vi "GenerateAnalogWaveformPiezoTraj.vi"(8 "error in (no error)":errorcluster, 11 "SetupInfo_IN":T1={"ConfigParameters_Analog"={"JAI camera fps"=240.0, "Bi-Lateral Galvo xy scan range (V)"=0.7, "Bi-Lateral Galvo xy scan frequency (Hz)"=500, "AOM Blind percent (%)"=0.1, "AOM start blind percent (%) "=70.0, "ROI threshold"=0.5, "AO Sampling rate"=1000000.0}, "ConfigParameters_Digital"={"Steps per volume"=25.0, "Time per volume (s)"=0.4, "OG start layer"=15.0, "Objective Lin Rising Vel (micron/ms）"=1.0, "Image depth (micron)"=200.0, "OG latency (s)"=10.0, "OG repitation"=3.0, "OG end layer"=17.0, "Shock1 duration (s)"=0.001, "Shock2 duration (s)"=0.001, "Shock3 duration (s)"=0.01, "Shock4 duration (s)"=0.01, "Shock5 duration (s)"=0.1, "Shock duration_New"=[]}, "ConfigParameters_Other1"={"Frontal Galvo xy scan range (V)"=0.14, "Frontal Galvo xy scan frequency (Hz)"=500, "PFI 0 digital clock frequency"=500000.0, "Window size for layer index"=0.5, "sCMOS fps"=95.0}, "ConfigParameters_Others2"={"#Trials baseline"=6, "#Trials test"=6, "Time before acq. (s)"=360.0, "Time before test (s)"=600.0, "#Blocks acquisition"=5, "Inter-trial interval baseline (s)"=60.0, "#Trials per acquition block"=6, "Inter-block interval acquisition (s)"=360.0, "Inter-trial interval acquisition (s)"=20.0, "Flash latency (s)"=10.0, "Flash duration (s)"=3.2, "Response duration (s)"=10.0, "MaxTimeEventDetection (s)"=6, "StimType"=enum."Flash", "#MaxEvents"=6}, "ProcessParametersOut"={"stand Z vol Acquisition time (s)"=0.2631578947368421, "stand Z vol Backward time (s)"=0.13684210526315793, "Objective scan volt"=5.0, "Bi-lateral Galvo Z scan volt"=0.45, "Frontal Galvo Z scan volt"=0.37, "Objective step length (micron)"=8.0, "OG Z volet Linear Dec time (s)"=0.024, "OG Z vol Stim. steps time (s)"=0.031578947368421054, "OG Z vol Linear Acc time (s)"=0.112, "#Vol. of flash"=8, "#Vol. of shock"=1, "#Vol. bef flash"=25, "#Vol. aft flash"=17, "OG Z vol Linear Dec time (s)"=0.112, "OG Z vol time (s)"=0.39073684210526316, "Stack duration"=[0.001, 0.001, 0.01, 0.01, 0.1], "AOM stand. value size"=400000, "Plane indexing length"=0, "#Vol. blank"=0, "#Vol. blank before acq"=0, "#Vol. blank before test"=0, " #Inter-block interval acquisition (Ed-St Vol)"=0}, "WaveformParameters"={"stand Z vol Acquisition samp info"={"Fs"=1000000.0, "#s"=263158.0}, "stand Z vol Backward samp info"={"Fs"=1000000.0, "#s"=136842.0}, "OG Z vol Linear Acc samp info"={"Fs"=1000000.0, "#s"=112000.0}, "OG Z vol Stim. steps samp info"={"Fs"=1000000.0, "#s"=31579.0}, "OG Z volet Linear Dec samp info"={"Fs"=1000000.0, "#s"=24000.0}, "OG Z vol Linear Dec samp info"={"Fs"=1000000.0, "#s"=112000.0}, "OG Z vol samp info"={"Fs"=1000000.0, "#s"=390737.0}, "stand Z vol backforth samp info"={"Fs"=1000000.0, "#s"=400000.0}}, "AnalogWaveform"={"Bi-lateral Galvo Z stand waveform"={"t0"=timestamp(0 s since 1904-01-01), "dt"=1.0, "Y"=[]}, "Frontal Galvo Z stand waveform"={"t0"=timestamp(0 s since 1904-01-01), "dt"=1.0, "Y"=[]}, "Bi-lateral Galvo XY stand waveform"={"t0"=timestamp(0 s since 1904-01-01), "dt"=1.0, "Y"=[]}, "Frontal Galvo XY stand waveform"={"t0"=timestamp(0 s since 1904-01-01), "dt"=1.0, "Y"=[]}, "sCMOS stand waveform"={"t0"=timestamp(0 s since 1904-01-01), "dt"=1.0, "Y"=[]}, "Detection objective stand waveform"={"t0"=timestamp(0 s since 1904-01-01), "dt"=1.0, "Y"=[]}, "AOM stand waveform"={"t0"=timestamp(0 s since 1904-01-01), "dt"=1.0, "Y"=[]}, "PFI 0 clock stand waveform"={"t0"=timestamp(0 s since 1904-01-01), "dt"=1.0, "Y"=[]}, "Bi-lateral Galvo Z OG waveform"={"t0"=timestamp(0 s since 1904-01-01), "dt"=1.0, "Y"=[]}, "Bi-lateral Galvo XY OG waveform"={"t0"=timestamp(0 s since 1904-01-01), "dt"=1.0, "Y"=[]}, "Frontal Galvo Z OG waveform"={"t0"=timestamp(0 s since 1904-01-01), "dt"=1.0, "Y"=[]}, "Frontal Galvo XY OG waveform"={"t0"=timestamp(0 s since 1904-01-01), "dt"=1.0, "Y"=[]}, "sCMOS OG waveform"={"t0"=timestamp(0 s since 1904-01-01), "dt"=1.0, "Y"=[]}, "Detection objective OG waveform"={"t0"=timestamp(0 s since 1904-01-01), "dt"=1.0, "Y"=[]}, "AOM OG waveform"={"t0"=timestamp(0 s since 1904-01-01), "dt"=1.0, "Y"=[]}, "PFI 0 clock OG wavee"={"t0"=timestamp(0 s since 1904-01-01), "dt"=1.0, "Y"=[]}, "sCMOS blank waveform"={"t0"=timestamp(0 s since 1904-01-01), "dt"=1.0, "Y"=[]}, "All analog OG wave"=[], "All analog stand wave"=[], "All analog blank wave"=[], "BufferWaveform_Analog"=[], "Bi-lateral Galvo Z XY"={"t0"=timestamp(0 s since 1904-01-01), "dt"=1.0, "Y"=[]}, "Frontal Galvo Z XY"={"t0"=timestamp(0 s since 1904-01-01), "dt"=1.0, "Y"=[]}, "sCMOS Trigger XY"={"t0"=timestamp(0 s since 1904-01-01), "dt"=1.0, "Y"=[]}, "Detection objective XY"={"t0"=timestamp(0 s since 1904-01-01), "dt"=1.0, "Y"=[]}, "AOM XY"={"t0"=timestamp(0 s since 1904-01-01), "dt"=1.0, "Y"=[]}, "Analog_XY"=[]}, "DigitalWaveform"={"AllDigitalStandWave"=[], "AllDigialEvokedWave"=[], "AllDigialOGWave"=[], "AllDigitalPairWave_1"=[], "AllDigitalPairWave_2"=[], "AllDigitalPairWave_3"=[], "AllDigitalPairWave_4"=[], "AllDigitalPairWave_5"=[], "Plane Indexing"={"t0"=timestamp(0 s since 1904-01-01), "dt"=0.0, "Y"={"transitions"=[], "data"=[]}, "error"={"status"=FALSE, "code"=37421928, "source"=""}}, "Plane indexing P0.5 OG"={"t0"=timestamp(0 s since 1904-01-01), "dt"=0.0, "Y"={"transitions"=[], "data"=[]}, "error"={"status"=FALSE, "code"=37421928, "source"=""}}, "AllDigitalPairWaves"=[], "BufferWaveform_Digital"=[], "AllDigitalBlankWave"=[], "Digial_XY"=[], "Digital_XY_flash"=[], "Digial_XY DMD"=[]}, "PhysicalResource"={"PhysicalChannels_AI"="", "PhysicalChannels_AO"="", "PhysicalChannels_DO"="", "Task_AnalogOutput"="", "Task_DigitalOutput"="", "Task_AnalogInput"=""}, "ControlsRef"={"Mode_1"=refnum, "EventDetectionMode"=refnum, "Mode_2A"=refnum, "StimulationMode"=refnum, "Mode_2B"=refnum, "ErrorMeg"=refnum}, "test"=""} {"ConfigParameters_Other1"."Frontal Galvo xy scan frequency (Hz)" min=500 max=500; "ConfigParameters_Other1"."Frontal Galvo xy scan range (V)" min=0.0 max=1.5; "ConfigParameters_Analog"."AOM start blind percent (%)" min=10.0 max=90.0; "ConfigParameters_Analog"."AOM Blind percent (%)" min=0.1 max=100.0; "ConfigParameters_Analog"."Bi-Lateral Galvo xy scan frequency (Hz)" min=500 max=500; "ConfigParameters_Analog"."Bi-Lateral Galvo xy scan range (V)" min=0.0 max=1.5}) -> (0 "error out":errorcluster, 3 "SetupInfo_OUT":T1={"ConfigParameters_Analog"={"JAI camera fps"=240.0, "Bi-Lateral Galvo xy scan range (V)"=0.7, "Bi-Lateral Galvo xy scan frequency (Hz)"=500, "AOM Blind percent (%)"=0.1, "AOM start blind percent (%) "=70.0, "ROI threshold"=1.0, "AO Sampling rate"=1000000.0}, "ConfigParameters_Digital"={"Steps per volume"=25.0, "Time per volume (s)"=0.4, "OG start layer"=15.0, "Objective Lin Rising Vel (micron/ms）"=1.0, "Image depth (micron)"=200.0, "OG latency (s)"=10.0, "OG repitation"=3.0, "OG end layer"=17.0, "Shock1 duration (s)"=0.001, "Shock2 duration (s)"=0.001, "Shock3 duration (s)"=0.01, "Shock4 duration (s)"=0.01, "Shock5 duration (s)"=0.1, "Shock duration_New"=[]}, "ConfigParameters_Other1"={"Frontal Galvo xy scan range (V)"=0.14, "Frontal Galvo xy scan frequency (Hz)"=500, "PFI 0 digital clock frequency"=500000.0, "Window size for layer index"=0.5, "sCMOS fps"=95.0}, "ConfigParameters_Others2"={"#Trials baseline"=6, "#Trials test"=6, "Time before acq. (s)"=360.0, "Time before test (s)"=600.0, "#Blocks acquisition"=5, "Inter-trial interval baseline (s)"=60.0, "#Trials per acquition block"=6, "Inter-block interval acquisition (s)"=360.0, "Inter-trial interval acquisition (s)"=20.0, "Flash latency (s)"=10.0, "Flash duration (s)"=3.2, "Response duration (s)"=10.0, "MaxTimeEventDetection (s)"=6, "StimType"=enum."Flash", "#MaxEvents"=6}, "ProcessParametersOut"={"stand Z vol Acquisition time (s)"=0.2631578947368421, "stand Z vol Backward time (s)"=0.13684210526315793, "Objective scan volt"=5.0, "Bi-lateral Galvo Z scan volt"=0.1800000180000018, "Frontal Galvo Z scan volt"=0.14940000509752818, "Objective step length (micron)"=8.0, "OG Z volet Linear Dec time (s)"=0.024, "OG Z vol Stim. steps time (s)"=0.031578947368421054, "OG Z vol Linear Acc time (s)"=0.112, "#Vol. of flash"=8, "#Vol. of shock"=1, "#Vol. bef flash"=25, "#Vol. aft flash"=17, "OG Z vol Linear Dec time (s)"=0.112, "OG Z vol time (s)"=0.39073684210526316, "Stack duration"=[0.001, 0.001, 0.01, 0.01, 0.1], "AOM stand. value size"=400000, "Plane indexing length"=0, "#Vol. blank"=0, "#Vol. blank before acq"=0, "#Vol. blank before test"=0, " #Inter-block interval acquisition (Ed-St Vol)"=0}, "WaveformParameters"={"stand Z vol Acquisition samp info"={"Fs"=1000000.0, "#s"=263158.0}, "stand Z vol Backward samp info"={"Fs"=1000000.0, "#s"=136842.0}, "OG Z vol Linear Acc samp info"={"Fs"=1000000.0, "#s"=112000.0}, "OG Z vol Stim. steps samp info"={"Fs"=1000000.0, "#s"=31579.0}, "OG Z volet Linear Dec samp info"={"Fs"=1000000.0, "#s"=24000.0}, "OG Z vol Linear Dec samp info"={"Fs"=1000000.0, "#s"=112000.0}, "OG Z vol samp info"={"Fs"=1000000.0, "#s"=390737.0}, "stand Z vol backforth samp info"={"Fs"=1000000.0, "#s"=400000.0}}, "AnalogWaveform"={"Bi-lateral Galvo Z stand waveform"={"t0"=timestamp(0 s since 1904-01-01), "dt"=1.0, "Y"=[]}, "Frontal Galvo Z stand waveform"={"t0"=timestamp(0 s since 1904-01-01), "dt"=1.0, "Y"=[]}, "Bi-lateral Galvo XY stand waveform"={"t0"=timestamp(0 s since 1904-01-01), "dt"=1.0, "Y"=[]}, "Frontal Galvo XY stand waveform"={"t0"=timestamp(0 s since 1904-01-01), "dt"=1.0, "Y"=[]}, "sCMOS stand waveform"={"t0"=timestamp(0 s since 1904-01-01), "dt"=1.0, "Y"=[]}, "Detection objective stand waveform"={"t0"=timestamp(0 s since 1904-01-01), "dt"=1.0, "Y"=[]}, "AOM stand waveform"={"t0"=timestamp(0 s since 1904-01-01), "dt"=1.0, "Y"=[]}, "PFI 0 clock stand waveform"={"t0"=timestamp(0 s since 1904-01-01), "dt"=1.0, "Y"=[]}, "Bi-lateral Galvo Z OG waveform"={"t0"=timestamp(0 s since 1904-01-01), "dt"=1.0, "Y"=[]}, "Bi-lateral Galvo XY OG waveform"={"t0"=timestamp(0 s since 1904-01-01), "dt"=1.0, "Y"=[]}, "Frontal Galvo Z OG waveform"={"t0"=timestamp(0 s since 1904-01-01), "dt"=1.0, "Y"=[]}, "Frontal Galvo XY OG waveform"={"t0"=timestamp(0 s since 1904-01-01), "dt"=1.0, "Y"=[]}, "sCMOS OG waveform"={"t0"=timestamp(0 s since 1904-01-01), "dt"=1.0, "Y"=[]}, "Detection objective OG waveform"={"t0"=timestamp(0 s since 1904-01-01), "dt"=1.0, "Y"=[]}, "AOM OG waveform"={"t0"=timestamp(0 s since 1904-01-01), "dt"=1.0, "Y"=[]}, "PFI 0 clock OG wavee"={"t0"=timestamp(0 s since 1904-01-01), "dt"=1.0, "Y"=[]}, "sCMOS blank waveform"={"t0"=timestamp(0 s since 1904-01-01), "dt"=1.0, "Y"=[]}, "All analog OG wave"=[], "All analog stand wave"=[], "All analog blank wave"=[], "BufferWaveform_Analog"=[], "Bi-lateral Galvo Z XY"={"t0"=timestamp(0 s since 1904-01-01), "dt"=1.0, "Y"=[]}, "Frontal Galvo Z XY"={"t0"=timestamp(0 s since 1904-01-01), "dt"=1.0, "Y"=[]}, "sCMOS Trigger XY"={"t0"=timestamp(0 s since 1904-01-01), "dt"=1.0, "Y"=[]}, "Detection objective XY"={"t0"=timestamp(0 s since 1904-01-01), "dt"=1.0, "Y"=[]}, "AOM XY"={"t0"=timestamp(0 s since 1904-01-01), "dt"=1.0, "Y"=[]}, "Analog_XY"=[]}, "DigitalWaveform"={"AllDigitalStandWave"=[], "AllDigialEvokedWave"=[], "AllDigialOGWave"=[], "AllDigitalPairWave_1"=[], "AllDigitalPairWave_2"=[], "AllDigitalPairWave_3"=[], "AllDigitalPairWave_4"=[], "AllDigitalPairWave_5"=[], "Plane Indexing"={"t0"=timestamp(0 s since 1904-01-01), "dt"=0.0, "Y"={"transitions"=[], "data"=[]}, "error"={"status"=FALSE, "code"=37421928, "source"=""}}, "Plane indexing P0.5 OG"={"t0"=timestamp(0 s since 1904-01-01), "dt"=0.0, "Y"={"transitions"=[], "data"=[]}, "error"={"status"=FALSE, "code"=37421928, "source"=""}}, "AllDigitalPairWaves"=[], "BufferWaveform_Digital"=[], "AllDigitalBlankWave"=[], "Digial_XY"=[], "Digital_XY_flash"=[], "Digial_XY DMD"=[]}, "PhysicalResource"={"PhysicalChannels_AI"="", "PhysicalChannels_AO"="", "PhysicalChannels_DO"="", "Task_AnalogOutput"="", "Task_DigitalOutput"="", "Task_AnalogInput"=""}, "ControlsRef"={"Mode_1"=refnum, "EventDetectionMode"=refnum, "Mode_2A"=refnum, "StimulationMode"=refnum, "Mode_2B"=refnum, "ErrorMeg"=refnum}, "test"=""} {"ConfigParameters_Other1"."Frontal Galvo xy scan frequency (Hz)" min=500 max=500; "ConfigParameters_Other1"."Frontal Galvo xy scan range (V)" min=0.0 max=1.5; "ConfigParameters_Analog"."AOM start blind percent (%)" min=10.0 max=90.0; "ConfigParameters_Analog"."AOM Blind percent (%)" min=0.1 max=100.0; "ConfigParameters_Analog"."Bi-Lateral Galvo xy scan frequency (Hz)" min=500 max=500; "ConfigParameters_Analog"."Bi-Lateral Galvo xy scan range (V)" min=0.0 max=1.5})   [LabVIEW 2018]
uses:
  SetupInfo.ctl
  ConfigParameters_Analog.ctl
  ConfigParameters_Digital.ctl
  ConfigParameters_Others1.ctl
  ConfigParameters_Others2.ctl
  ProcessParametersOut.ctl
  WaveformParameters.ctl
  AnalogWaveform.ctl
  DigitalWaveform.ctl
  PhysicalResource.ctl
  ControlsRef.ctl
  <vilib>/Waveform/WDTOps.llb/WDT Append Waveforms DBL.vi
  <vilib>/measure/NI_MABase.lvlib
panel:
  out "piezo trajectory not in use. the trajactory version save in *copy.vi":string
  in  "FileSamplingRate":dbl=1000.0
  in  "PiezoTrajectoryPath":path=path "D:/APP/LightSheetController_Ver8 obl/VISource/Waveform/Piezo_feedback_20201106.txt"
  out "AOM stand. value size":i32=400000
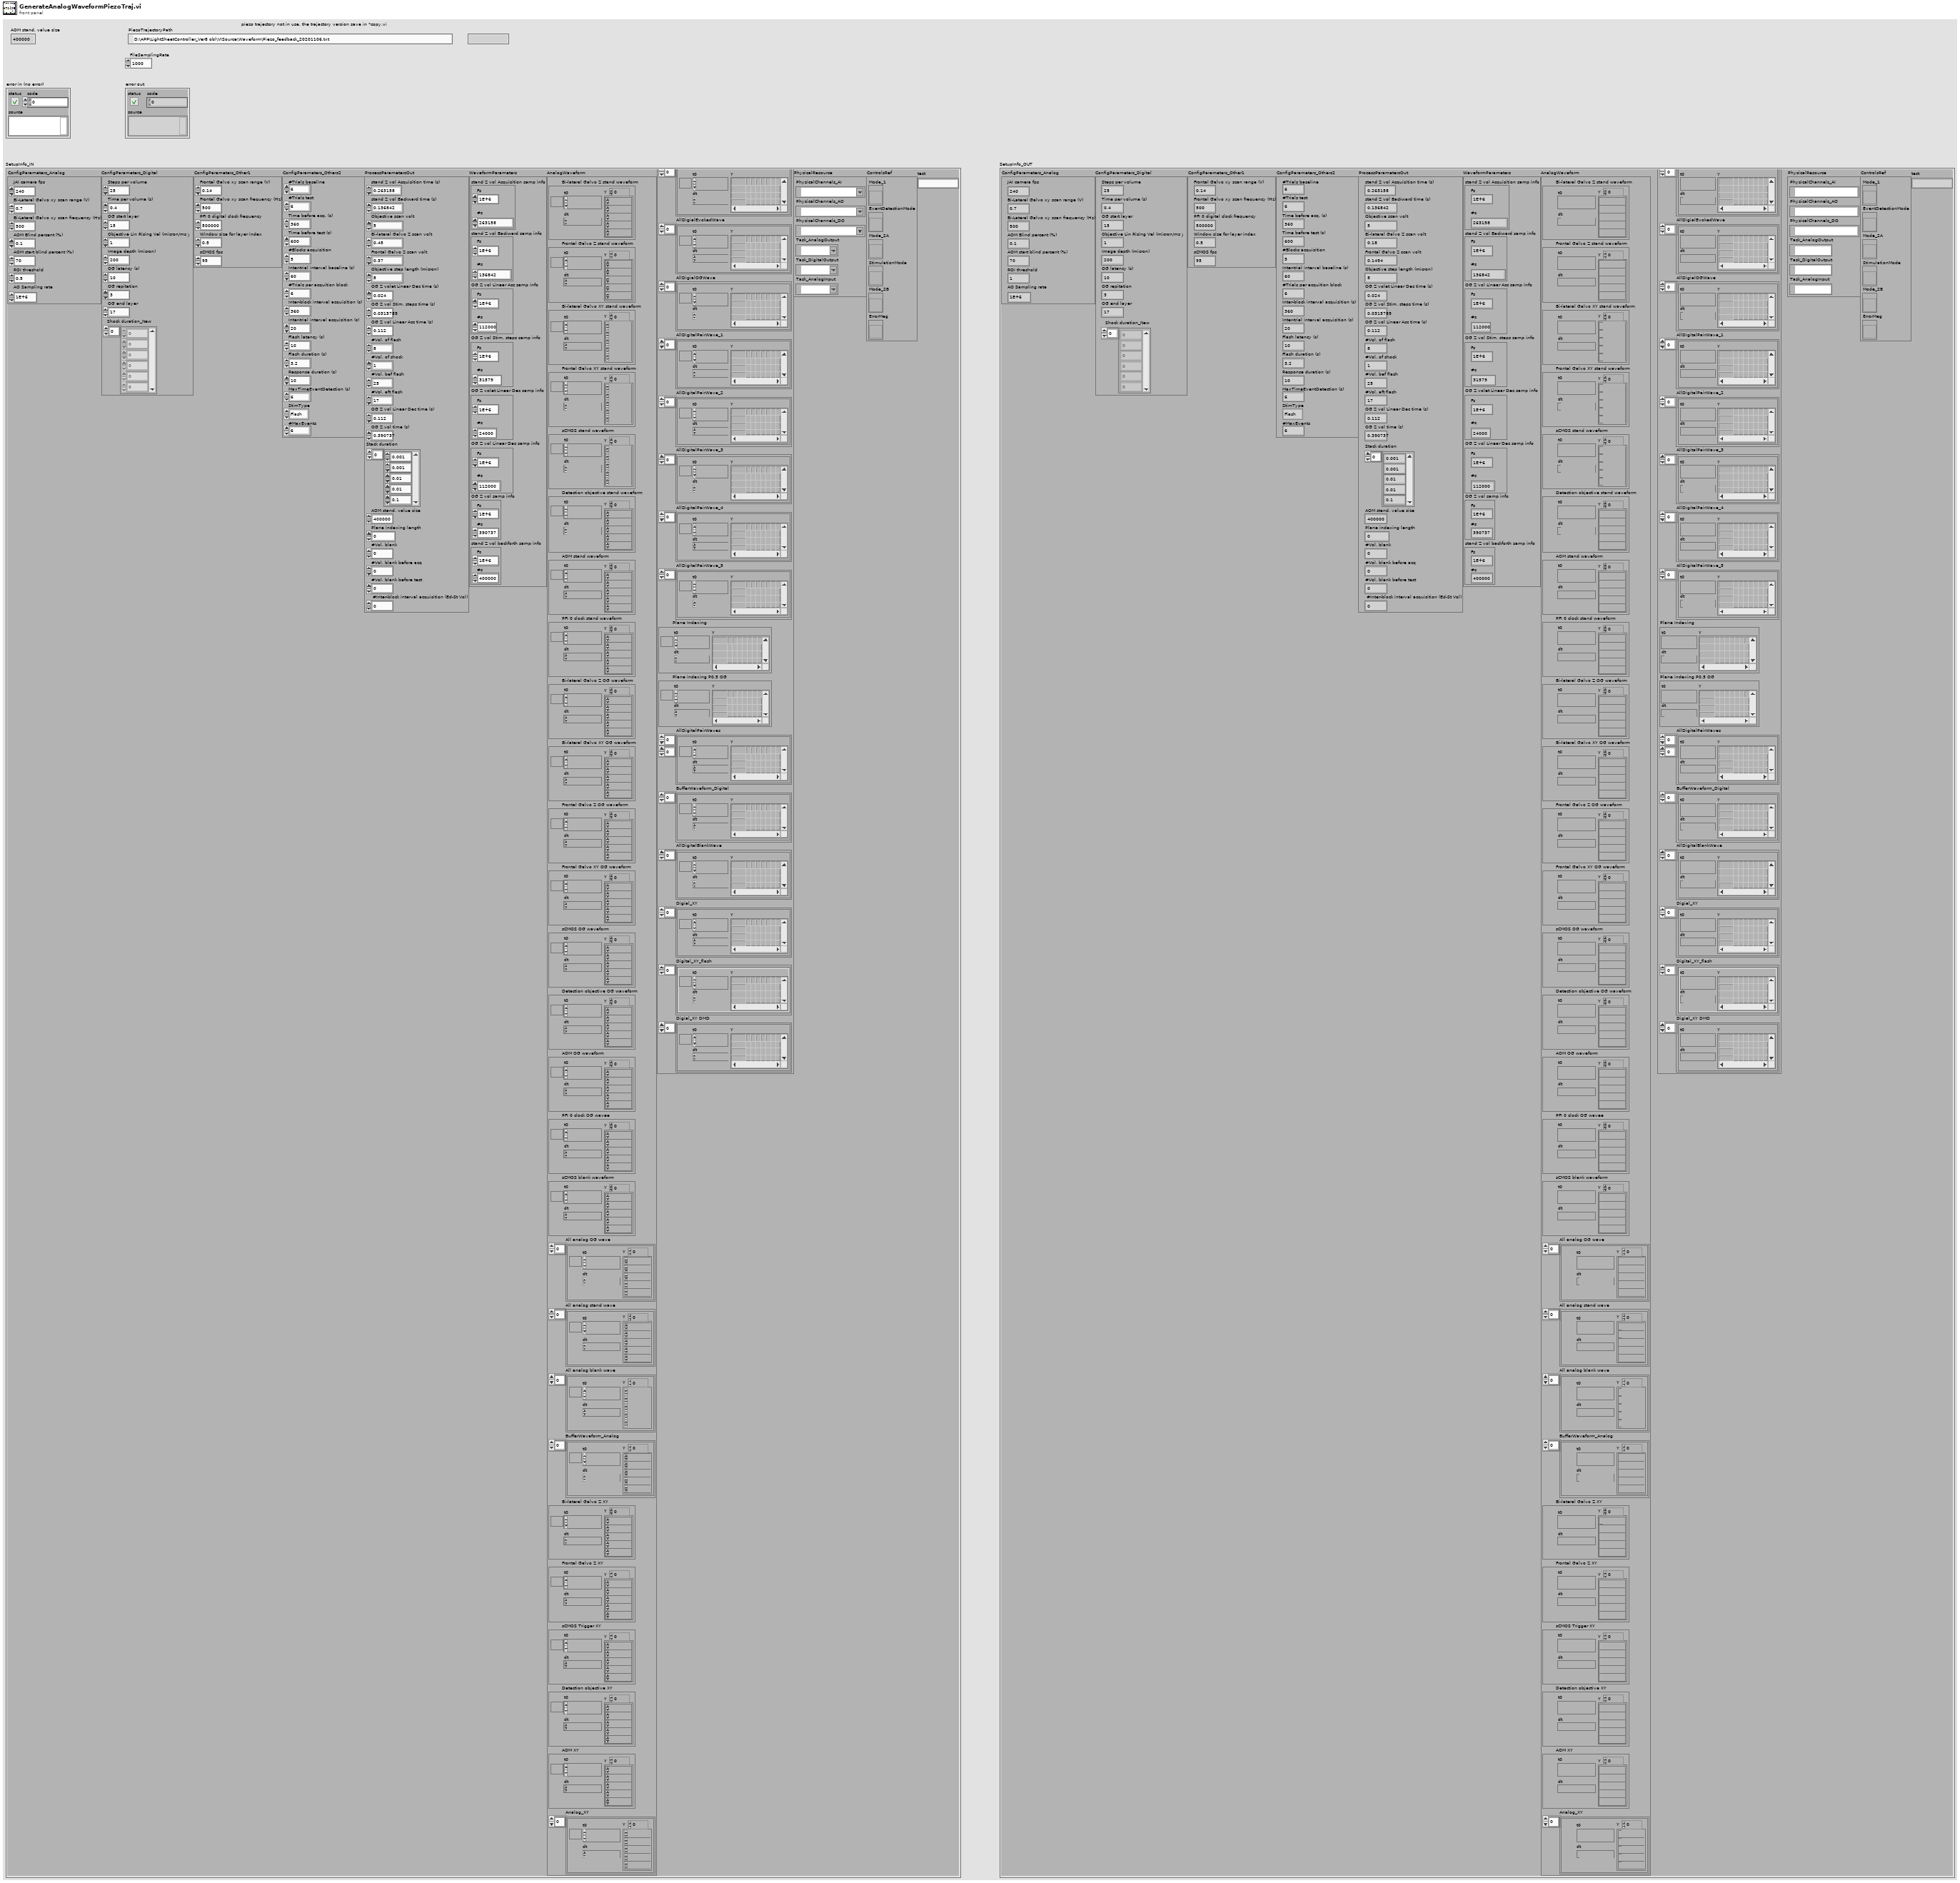
[diagram p1: front panel]
types:
  T1 = typedef "SetupInfo.ctl" = cluster{"ConfigParameters_Analog":T2, "ConfigParameters_Digital":T3, "ConfigParameters_Other1":T4, "ConfigParameters_Others2":T5, "ProcessParametersOut":T6, "WaveformParameters":T7, "AnalogWaveform":T8, "DigitalWaveform":T9, "PhysicalResource":T10, "ControlsRef":T11, "test":string}
  T2 = typedef "ConfigParameters_Analog.ctl" = cluster{"JAI camera fps":dbl, "Bi-Lateral Galvo xy scan range (V)":dbl, "Bi-Lateral Galvo xy scan frequency (Hz)":i16, "AOM Blind percent (%)":dbl, "AOM start blind percent (%) ":dbl, "ROI threshold":dbl, "AO Sampling rate":dbl}
  T3 = typedef "ConfigParameters_Digital.ctl" = cluster{"Steps per volume":dbl, "Time per volume (s)":dbl, "OG start layer":dbl, "Objective Lin Rising Vel (micron/ms）":dbl, "Image depth (micron)":dbl, "OG latency (s)":dbl, "OG repitation":dbl, "OG end layer":dbl, "Shock1 duration (s)":dbl, "Shock2 duration (s)":dbl, "Shock3 duration (s)":dbl, "Shock4 duration (s)":dbl, "Shock5 duration (s)":dbl, "Shock duration_New":dbl[]}
  T4 = typedef "ConfigParameters_Others1.ctl" = cluster{"Frontal Galvo xy scan range (V)":dbl, "Frontal Galvo xy scan frequency (Hz)":i16, "PFI 0 digital clock frequency":dbl, "Window size for layer index":dbl, "sCMOS fps":dbl}
  T5 = typedef "ConfigParameters_Others2.ctl" = cluster{"#Trials baseline":i32, "#Trials test":i32, "Time before acq. (s)":dbl, "Time before test (s)":dbl, "#Blocks acquisition":i32, "Inter-trial interval baseline (s)":dbl, "#Trials per acquition block":i32, "Inter-block interval acquisition (s)":dbl, "Inter-trial interval acquisition (s)":dbl, "Flash latency (s)":dbl, "Flash duration (s)":dbl, "Response duration (s)":dbl, "MaxTimeEventDetection (s)":i32, "StimType":enum16{"Flash", "OG"}, "#MaxEvents":i32}
  T6 = typedef "ProcessParametersOut.ctl" = cluster{"stand Z vol Acquisition time (s)":dbl, "stand Z vol Backward time (s)":dbl, "Objective scan volt":dbl, "Bi-lateral Galvo Z scan volt":dbl, "Frontal Galvo Z scan volt":dbl, "Objective step length (micron)":dbl, "OG Z volet Linear Dec time (s)":dbl, "OG Z vol Stim. steps time (s)":dbl, "OG Z vol Linear Acc time (s)":dbl, "#Vol. of flash":i32, "#Vol. of shock":i32, "#Vol. bef flash":i32, "#Vol. aft flash":i32, "OG Z vol Linear Dec time (s)":dbl, "OG Z vol time (s)":dbl, "Stack duration":dbl[], "AOM stand. value size":i32, "Plane indexing length":i32, "#Vol. blank":i32, "#Vol. blank before acq":i32, "#Vol. blank before test":i32, " #Inter-block interval acquisition (Ed-St Vol)":i32}
  T7 = typedef "WaveformParameters.ctl" = cluster{"stand Z vol Acquisition samp info":cluster{"Fs":dbl, "#s":dbl}, "stand Z vol Backward samp info":cluster{"Fs":dbl, "#s":dbl}, "OG Z vol Linear Acc samp info":cluster{"Fs":dbl, "#s":dbl}, "OG Z vol Stim. steps samp info":cluster{"Fs":dbl, "#s":dbl}, "OG Z volet Linear Dec samp info":cluster{"Fs":dbl, "#s":dbl}, "OG Z vol Linear Dec samp info":cluster{"Fs":dbl, "#s":dbl}, "OG Z vol samp info":cluster{"Fs":dbl, "#s":dbl}, "stand Z vol backforth samp info":cluster{"Fs":dbl, "#s":dbl}}
  T8 = typedef "AnalogWaveform.ctl" = cluster{"Bi-lateral Galvo Z stand waveform":waveform(dbl), "Frontal Galvo Z stand waveform":waveform(dbl), "Bi-lateral Galvo XY stand waveform":waveform(dbl), "Frontal Galvo XY stand waveform":waveform(dbl), "sCMOS stand waveform":waveform(dbl), "Detection objective stand waveform":waveform(dbl), "AOM stand waveform":waveform(dbl), "PFI 0 clock stand waveform":waveform(dbl), "Bi-lateral Galvo Z OG waveform":waveform(dbl), "Bi-lateral Galvo XY OG waveform":waveform(dbl), "Frontal Galvo Z OG waveform":waveform(dbl), "Frontal Galvo XY OG waveform":waveform(dbl), "sCMOS OG waveform":waveform(dbl), "Detection objective OG waveform":waveform(dbl), "AOM OG waveform":waveform(dbl), "PFI 0 clock OG wavee":waveform(dbl), "sCMOS blank waveform":waveform(dbl), "All analog OG wave":waveform(dbl)[], "All analog stand wave":waveform(dbl)[], "All analog blank wave":waveform(dbl)[], "BufferWaveform_Analog":waveform(dbl)[], "Bi-lateral Galvo Z XY":waveform(dbl), "Frontal Galvo Z XY":waveform(dbl), "sCMOS Trigger XY":waveform(dbl), "Detection objective XY":waveform(dbl), "AOM XY":waveform(dbl), "Analog_XY":waveform(dbl)[]}
  T9 = typedef "DigitalWaveform.ctl" = cluster{"AllDigitalStandWave":digitalwaveform[], "AllDigialEvokedWave":digitalwaveform[], "AllDigialOGWave":digitalwaveform[], "AllDigitalPairWave_1":digitalwaveform[], "AllDigitalPairWave_2":digitalwaveform[], "AllDigitalPairWave_3":digitalwaveform[], "AllDigitalPairWave_4":digitalwaveform[], "AllDigitalPairWave_5":digitalwaveform[], "Plane Indexing":digitalwaveform, "Plane indexing P0.5 OG":digitalwaveform, "AllDigitalPairWaves":digitalwaveform[][], "BufferWaveform_Digital":digitalwaveform[], "AllDigitalBlankWave":digitalwaveform[], "Digial_XY":digitalwaveform[], "Digital_XY_flash":digitalwaveform[], "Digial_XY DMD":digitalwaveform[]}
  T10 = typedef "PhysicalResource.ctl" = cluster{"PhysicalChannels_AI":tag, "PhysicalChannels_AO":tag, "PhysicalChannels_DO":tag, "Task_AnalogOutput":refnum<k21>, "Task_DigitalOutput":refnum<k21>, "Task_AnalogInput":refnum<k21>}
  T11 = typedef "ControlsRef.ctl" = cluster{"Mode_1":refnum<vi>, "EventDetectionMode":refnum<vi>, "Mode_2A":refnum<vi>, "StimulationMode":refnum<vi>, "Mode_2B":refnum<vi>, "ErrorMeg":refnum<vi>}
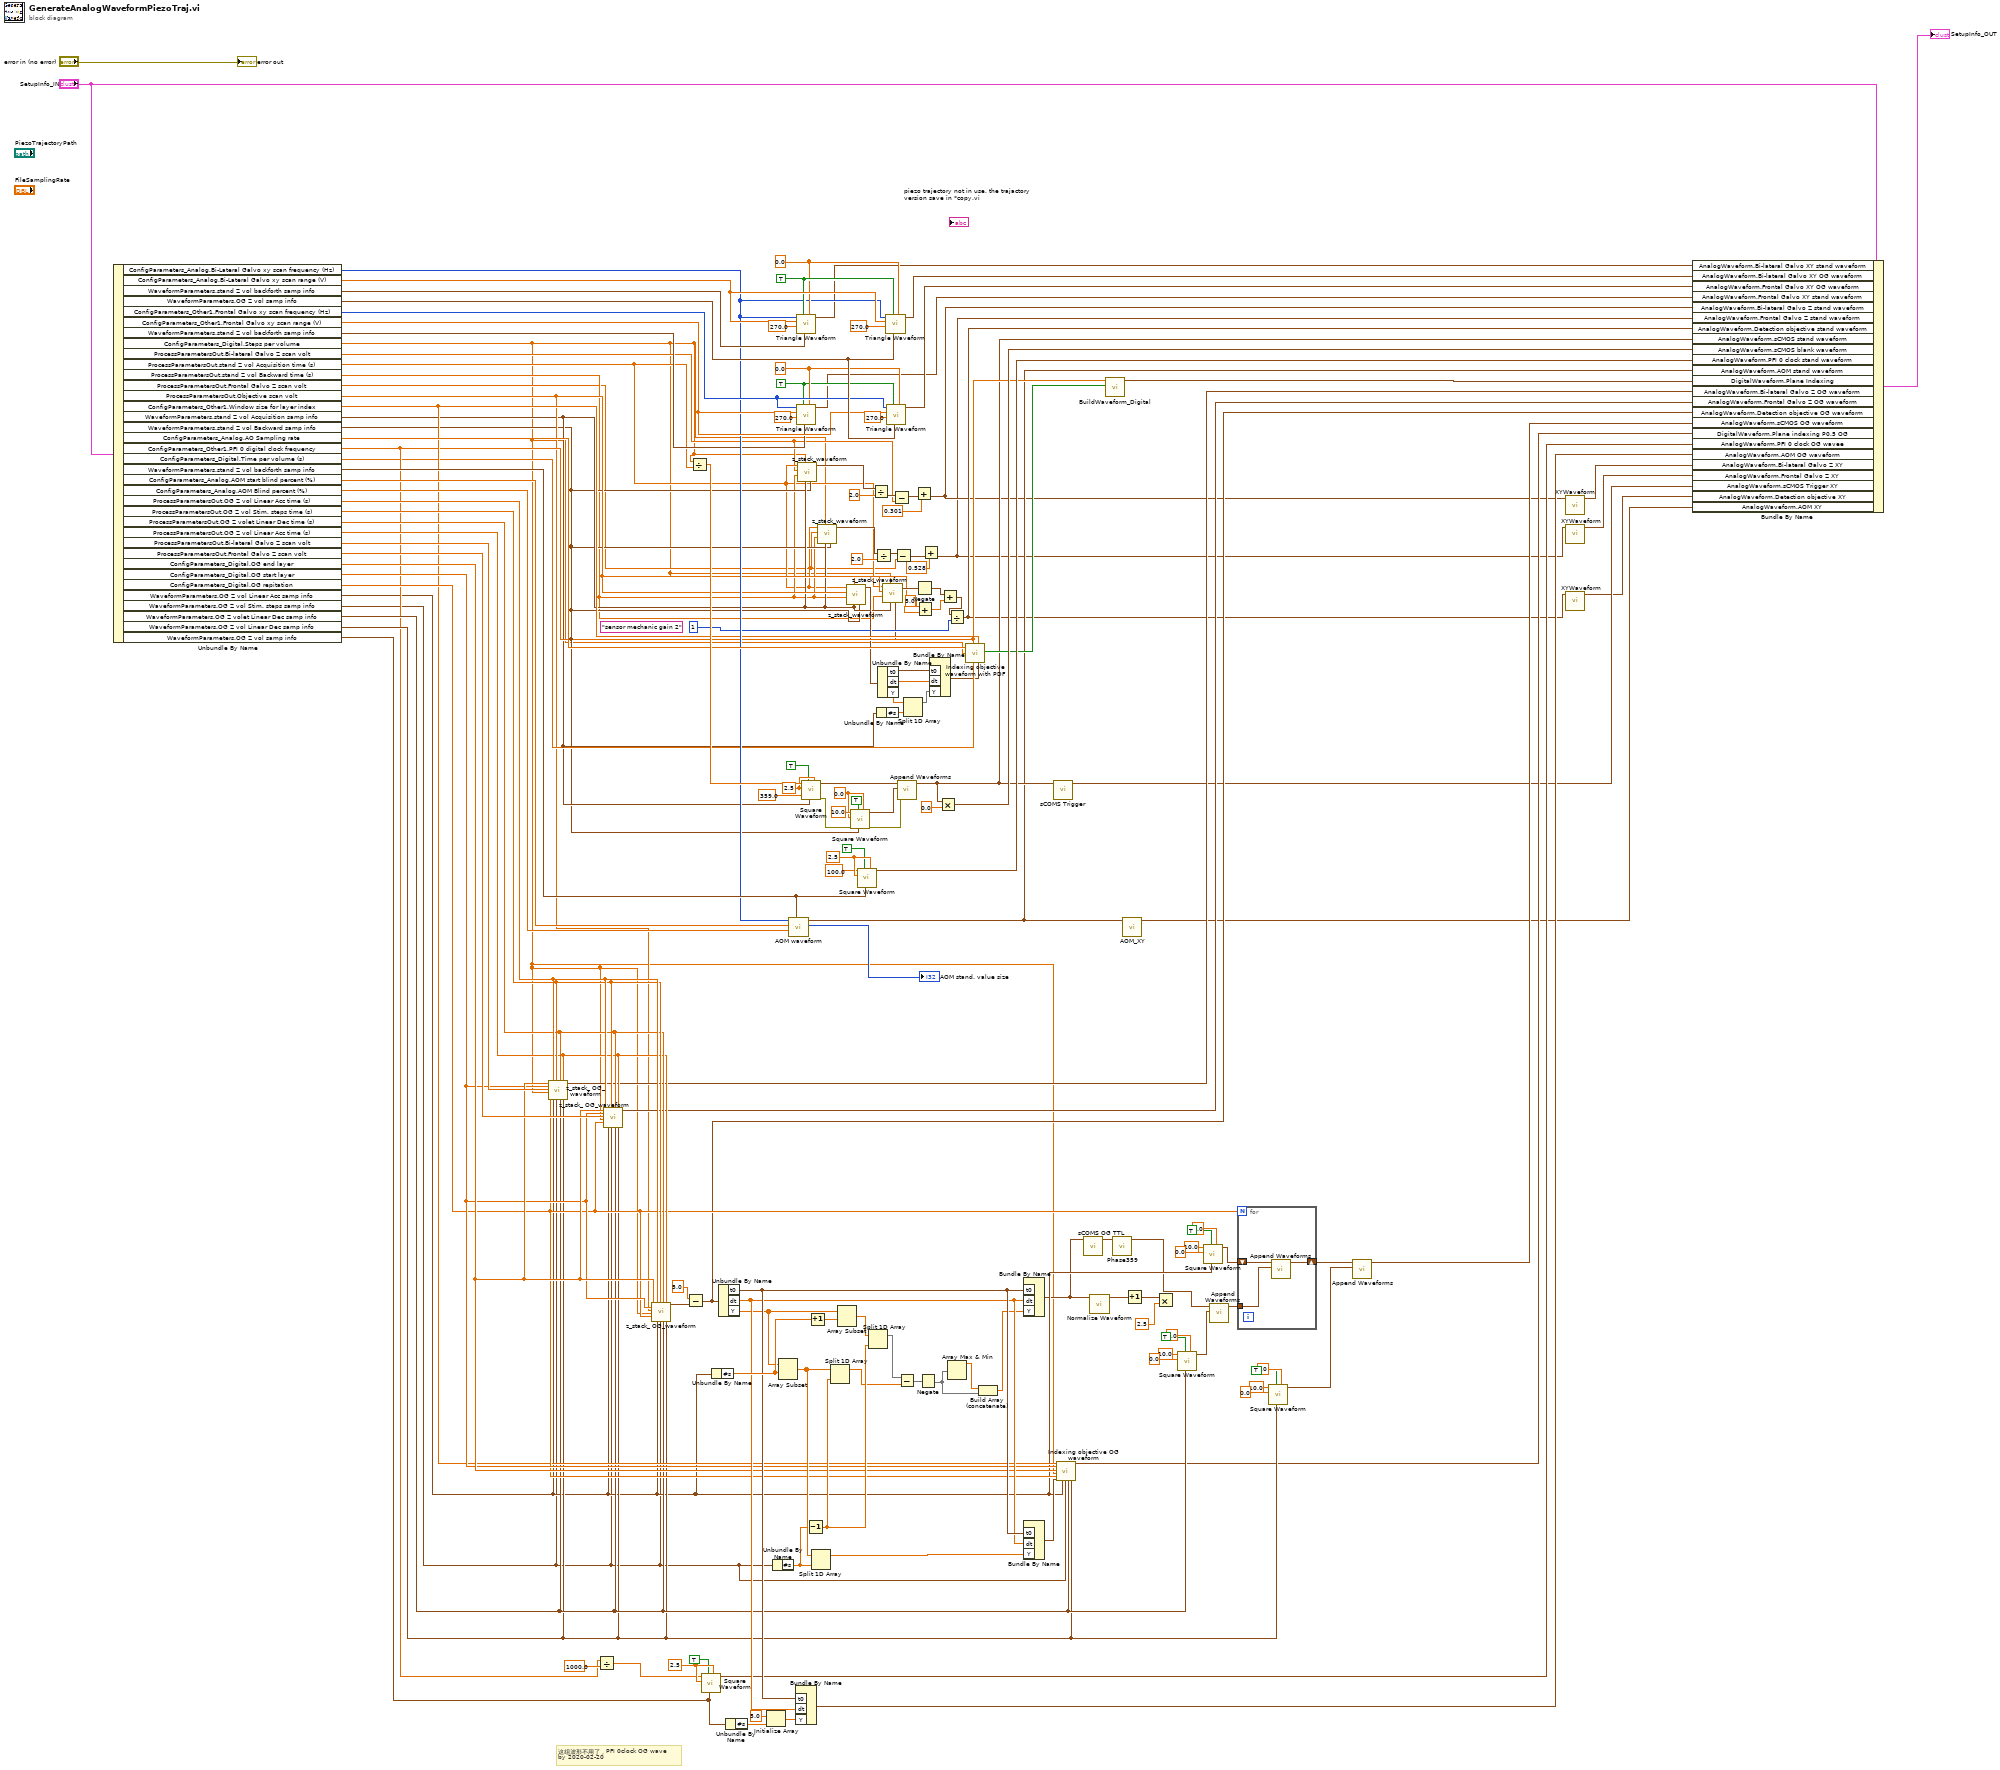
[diagram p0: block diagram]
diagram:
  (unwired) "sensor mechanic gain 2"
  w90 = 2.5
  w135 = 2.5 ("offset")
  w142 = 0.0 ("offset")
  w146 = 2.5 ("amplitude")
  w121 = TRUE ("reset signal")
  w129 = TRUE ("reset signal")
  w128 = 0.0 ("offset")
  w122 = 0.0 ("offset")
  # "这组波形不用了，PFI 0clock OG wave\nby 2020-02-20"
  n1 = Unbundle By Name("SetupInfo_IN") -> ("ConfigParameters_Analog.Bi-Lateral Galvo xy scan frequency (Hz)"=w117:i16, "ConfigParameters_Analog.Bi-Lateral Galvo xy scan range (V)"=w131:dbl, "WaveformParameters.stand Z vol backforth samp info"=w130:cluster{"Fs":dbl, "#s":dbl}, "WaveformParameters.OG Z vol samp info"=w126:cluster{"Fs":dbl, "#s":dbl}, "ConfigParameters_Other1.Frontal Galvo xy scan frequency (Hz)"=w125:i16, "ConfigParameters_Other1.Frontal Galvo xy scan range (V)"=w124:dbl, "WaveformParameters.stand Z vol backforth samp info"=w23:cluster{"Fs":dbl, "#s":dbl}, "ConfigParameters_Digital.Steps per volume"=w1:dbl, "ProcessParametersOut.Bi-lateral Galvo Z scan volt"=w3:dbl, "ProcessParametersOut.stand Z vol Acquisition time (s)"=w4:dbl, "ProcessParametersOut.stand Z vol Backward time (s)"=w5:dbl, "ProcessParametersOut.Frontal Galvo Z scan volt"=w2:dbl, "ProcessParametersOut.Objective scan volt"=w20:dbl, "ConfigParameters_Other1.Window size for layer index"=w74:dbl, "WaveformParameters.stand Z vol Acquisition samp info"=w7:cluster{"Fs":dbl, "#s":dbl}, "WaveformParameters.stand Z vol Backward samp info"=w6:cluster{"Fs":dbl, "#s":dbl}, "ConfigParameters_Analog.AO Sampling rate"=w119:dbl, "ConfigParameters_Other1.PFI 0 digital clock frequency"=w58:dbl, "ConfigParameters_Digital.Time per volume (s)"=w57:dbl, "WaveformParameters.stand Z vol backforth samp info"=w118:cluster{"Fs":dbl, "#s":dbl}, "ConfigParameters_Analog.AOM start blind percent (%)"=w116:dbl, "ConfigParameters_Analog.AOM Blind percent (%)"=w115:dbl, "ProcessParametersOut.OG Z vol Linear Acc time (s)"=w83:dbl, "ProcessParametersOut.OG Z vol Stim. steps time (s)"=w82:dbl, "ProcessParametersOut.OG Z volet Linear Dec time (s)"=w81:dbl, "ProcessParametersOut.OG Z vol Linear Acc time (s)"=w80:dbl, "ProcessParametersOut.Bi-lateral Galvo Z scan volt"=w79:dbl, "ProcessParametersOut.Frontal Galvo Z scan volt"=w78:dbl, "ConfigParameters_Digital.OG end layer"=w77:dbl, "ConfigParameters_Digital.OG start layer"=w76:dbl, "ConfigParameters_Digital.OG repitation"=w75:dbl, "WaveformParameters.OG Z vol Linear Acc samp info"=w40:cluster{"Fs":dbl, "#s":dbl}, "WaveformParameters.OG Z vol Stim. steps samp info"=w39:cluster{"Fs":dbl, "#s":dbl}, "WaveformParameters.OG Z volet Linear Dec samp info"=w73:cluster{"Fs":dbl, "#s":dbl}, "WaveformParameters.OG Z vol Linear Dec samp info"=w72:cluster{"Fs":dbl, "#s":dbl}, "WaveformParameters.OG Z vol samp info"=w71:cluster{"Fs":dbl, "#s":dbl})
  n2 = call "z_stack_ OG_waveform.vi"("OG end layer"=w77, "OG start layer"=w76, "SPECIFIC scan volt"=w79, "Steps per volume"=w1, "OG repitation"=w75, "Objective线性加速时间"=w83, "OG Z stack 线性加速 采样信息"=w40, "Objective 刺激steps 时间（s）"=w82, "OG Z stack 刺激steps 采样信息"=w39, "Objective volet 线性减速 时间（s）"=w81, "OG Z volet 线性减速 采样信息"=w73, "Objective线性减速时间"=w80, "OG Z stack 线性减速 采样信息"=w72) -> ("waveform out"=w61:waveform(dbl))  [unwired: 2 in, 4 out]
  n3 = Divide(x=w58, y=1000.0) -> (x/y=w64:dbl)
  n4 = call "z_stack_ OG_waveform.vi"("OG end layer"=w77, "OG start layer"=w76, "SPECIFIC scan volt"=w78, "Steps per volume"=w1, "OG repitation"=w75, "Objective线性加速时间"=w83, "OG Z stack 线性加速 采样信息"=w40, "Objective 刺激steps 时间（s）"=w82, "OG Z stack 刺激steps 采样信息"=w39, "Objective volet 线性减速 时间（s）"=w81, "OG Z volet 线性减速 采样信息"=w73, "Objective线性减速时间"=w80, "OG Z stack 线性减速 采样信息"=w72) -> ("waveform out"=w60:waveform(dbl))  [unwired: 2 in, 4 out]
  n5 = call "z_stack_ OG_waveform.vi"("OG end layer"=w77, "OG start layer"=w76, "SPECIFIC scan volt"=w20, "Steps per volume"=w1, "OG repitation"=w75, "Objective线性加速时间"=w83, "OG Z stack 线性加速 采样信息"=w40, "Objective 刺激steps 时间（s）"=w82, "OG Z stack 刺激steps 采样信息"=w39, "Objective volet 线性减速 时间（s）"=w81, "OG Z volet 线性减速 采样信息"=w73, "Objective线性减速时间"=w80, "OG Z stack 线性减速 采样信息"=w72) -> ("waveform out"=w53:waveform(dbl))  [unwired: 2 in, 4 out]
  n6 = Subtract(x=5.0, y=w53) -> (x-y=w48:waveform(dbl))
  n7 = Divide(x=w1, y=w4) -> (x/y=w147:dbl)
  n8 = call <vilib>:"Square Waveform.vi"("offset"=w90, "sampling info"=w71, "reset signal"=TRUE, "amplitude"=w90, "frequency"=w64) -> ("signal out"=w69:waveform(dbl))  [unwired: 5 in, 1 out]
  n9 = Unbundle By Name(w40) -> ("#s"=w91:dbl)
  n10 = Unbundle By Name(w48) -> ("t0"=w86:timestamp, "dt"=w85:dbl, "Y"=w51:dbl[])
  n11 = Unbundle By Name(w71) -> ("#s"=w84:dbl)
  n12 = Initialize Array(5.0 ("element"), w84) -> (w87:dbl[])
  n13 = Unbundle By Name(w39) -> ("#s"=w92:dbl)
  n14 = Array Subset(array=w51, index=w91) -> (w108:dbl[])  [unwired: 1 in]
  n15 = call "AOM waveform.vi"("z stack 往复采样信息"=w118, "AOM Blind percent (%)"=w115, "AOM start blind percent (%)"=w116, "Bi-Lateral Galvo xy scan frequency (Hz)"=w117) -> ("数值"=→"AOM stand. value size":i32, "Waveform"=w27:waveform(dbl))  [unwired: 6 in]
  n16 = Bundle By Name("t0"=w86, "dt"=w85, "Y"=w87) -> (w68:waveform(dbl))  [unwired: 1 in]
  n17 = call <vilib>:"Triangle Waveform.vi"("offset"=w128, "sampling info"=w130, "reset signal"=w129, "phase"=270.0, "amplitude"=w131, "frequency"=w117) -> ("signal out"=w66:waveform(dbl))  [unwired: 4 in, 1 out]
  n18 = call <vilib>:"Triangle Waveform.vi"("offset"=w122, "sampling info"=w23, "reset signal"=w121, "phase"=270.0, "amplitude"=w124, "frequency"=w125) -> ("signal out"=w120:waveform(dbl))  [unwired: 4 in, 1 out]
  n19 = call "z_stack_waveform.vi"("Z stack backward"=w6, "Z stack acquisition"=w7, "Steps per Volume"=w1, "Backward Time (s)"=w5, "SPECIFIC scan volt"=w3, "Aquisition Time (s)"=w4) -> ("WaveformOut"=w9:waveform(dbl))  [unwired: 5 in]
  n20 = call <vilib>:"Square Waveform.vi"("offset"=w146, "sampling info"=w7, "reset signal"=TRUE, "phase"=359.0, "amplitude"=w146, "frequency"=w147) -> ("error out"=w140:errorcluster, "signal out"=w138:waveform(dbl))  [unwired: 4 in]
  n21 = Decrement(x=w92) -> (x-1=w109:dbl)
  n22 = Increment(x=w91) -> (x+1=w110:dbl)
  n23 = Split 1D Array(array=w108, index=w92) -> (first subarray=w107:dbl[])  [unwired: 1 out]
  n24 = call "z_stack_waveform.vi"("Z stack backward"=w6, "Z stack acquisition"=w7, "Steps per Volume"=w1, "Backward Time (s)"=w5, "SPECIFIC scan volt"=w2, "Aquisition Time (s)"=w4) -> ("WaveformOut"=w8:waveform(dbl))  [unwired: 5 in]
  n25 = Split 1D Array(array=w108, index=w109) -> (first subarray=w44:dbl[])  [unwired: 1 out]
  n26 = Array Subset(array=w51, index=w110) -> (w50:dbl[])  [unwired: 1 in]
  n27 = call "z_stack_waveform.vi"("Z stack backward"=w6, "Z stack acquisition"=w7, "Steps per Volume"=w1, "Backward Time (s)"=w5, "SPECIFIC scan volt"=w20, "Aquisition Time (s)"=w4) -> ("WaveformOut"=w55:waveform(dbl))  [unwired: 5 in]
  n28 = call <vilib>:"Square Waveform.vi"("offset"=w142, "sampling info"=w6, "reset signal"=TRUE, "error in (no error)"=w140, "amplitude"=w142, "frequency"=10.0) -> ("error out"=w137:errorcluster, "signal out"=w139:waveform(dbl))  [unwired: 4 in]
  n29 = call <vilib>:"Square Waveform.vi"("offset"=w135, "sampling info"=w118, "reset signal"=TRUE, "amplitude"=w135, "frequency"=100.0 ("amplitude")) -> ("signal out"=w113:waveform(dbl))  [unwired: 5 in, 1 out]
  n30 = Split 1D Array(array=w50, index=w109) -> (first subarray=w45:dbl[])  [unwired: 1 out]
  n31 = Divide(x=w9, y=2.0) -> (x/y=w17:waveform(dbl))
  n32 = Divide(x=w8, y=2.0) -> (x/y=w15:waveform(dbl))
  n33 = Unbundle By Name(w7) -> ("#s"=w149:dbl)
  n34 = Unbundle By Name(w55) -> ("t0"=w152:timestamp, "dt"=w151:dbl, "Y"=w150:dbl[])
  n35 = call "z_stack_waveform.vi"("Z stack backward"=w6, "Z stack acquisition"=w7, "Steps per Volume"=w1, "Backward Time (s)"=w5, "SPECIFIC scan volt"=w20, "Aquisition Time (s)"=w4) -> ("WaveformOut"=w26:waveform(dbl))  [unwired: 5 in]
  n36 = call <vilib>:"Triangle Waveform.vi"("offset"=w128, "sampling info"=w126, "reset signal"=w129, "phase"=270.0, "amplitude"=w131, "frequency"=w117) -> ("signal out"=w127:waveform(dbl))  [unwired: 4 in, 1 out]
  n37 = call <vilib>:"Triangle Waveform.vi"("offset"=w122, "sampling info"=w126, "reset signal"=w121, "phase"=270.0, "amplitude"=w124, "frequency"=w125) -> ("signal out"=w123:waveform(dbl))  [unwired: 4 in, 1 out]
  n38 = Subtract(x=w17, y=w3) -> (x-y=w18:waveform(dbl))
  n39 = Subtract(x=w15, y=w2) -> (x-y=w19:waveform(dbl))
  n40 = call-poly <vilib>:"Append Waveforms.vi"("error in (no error)"=w137, "waveform B"=w139, "waveform A"=w138) -> ("waveform out"=w31:waveform(dbl))  [unwired: 7 in, 1 out]
  n41 = Subtract(x=w45, y=w44) -> (x-y=w42:dbl[])
  n42 = Split 1D Array(array=w150, index=w149) -> (first subarray=w148:dbl[])  [unwired: 1 out]
  n43 = Add(x=0.301, y=w18) -> (x+y=w13:waveform(dbl))
  n44 = Negate(x=w26) -> (-x=w154:waveform(dbl))
  n45 = Add(x=5.0, y=w20) -> (x+y=w153:dbl)
  n46 = Negate(x=w42) -> (-x=w49:dbl[])
  n47 = Add(x=0.528, y=w19) -> (x+y=w12:waveform(dbl))
  n48 = Bundle By Name("t0"=w152, "dt"=w151, "Y"=w148) -> (w56:waveform(dbl))  [unwired: 1 in]
  n49 = Multiply(x=w31, y=0.0) -> (x*y=w114:waveform(dbl))
  n50 = Add(x=w154, y=w153) -> (x+y=w25:waveform(dbl))
  n51 = Divide(x=w25, y=1) -> (x/y=w24:waveform(dbl))
  n52 = Array Max & Min(array=w49) -> (max value=w111:dbl)  [unwired: 3 out]
  n53 = call "Indexing objective waveform with PDF.vi"("AO sampling rate"=w119, "PFI0 digital clock frequency"=w58, "Steps per Volume"=w1, "Time per volume (s)"=w57, "Window size for layer index (ms)"=w74, "Steps Waveform"=w56) -> ("Plane Indexing data"=w63:bool[])  [unwired: 3 in, 1 out]
  n54 = Build Array (concatenate)(w111, w49) -> (w41:dbl[])
  n55 = Bundle By Name("t0"=w86, "dt"=w85, "Y"=w41) -> (w37:waveform(dbl))  [unwired: 1 in]
  n56 = Bundle By Name("t0"=w86, "dt"=w85, "Y"=w107) -> (w106:waveform(dbl))  [unwired: 1 in]
  n57 = call "sCOMS Trigger.vi"("In"=w31) -> ("Out"=w30:waveform(dbl))  [unwired: 10 in]
  n58 = call "Indexing objective OG waveform.vi"("Window size for layer index"=w74, "OG start layer"=w76, "OG end layer"=w77, "Steps per Volume"=w1, "OG repitation"=w75, "Waveform"=w106, "OG Z 线性加速 采样信息"=w40, "OG Z stack 刺激 steps 采样信息"=w39, "OG Z volet 线性减速 采样信息"=w73, "OG Z 线性减速 采样信息"=w72) -> ("Waveform_Digital"=w70:digitalwaveform)  [unwired: 9 in]
  n59 = call "sCOMS OG TTL.vi"("DataIn"=w37) -> ("Out"=w35:waveform(dbl))  [unwired: 10 in]
  n60 = call <vilib>:"Normalize Waveform.vi"("waveform in"=w37) -> ("normalized waveform"=w52:waveform(dbl))  [unwired: 7 in, 3 out]
  n61 = call "BuildWaveform_Digital.vi"("DigitalData"=w63, "SampleRate"=w58) -> ("DigitalWaveformOut"=w59:digitalwaveform)  [unwired: 9 in]
  n62 = call "Phase359.vi"("DataIn"=w35) -> ("DataOut"=w34:waveform(dbl))  [unwired: 10 in]
  n63 = call "AOM_XY.vi"("In"=w27) -> ("Out"=w28:waveform(dbl))  [unwired: 10 in]
  n64 = Increment(x=w52) -> (x+1=w54:waveform(dbl))
  n65 = Multiply(x=w54, y=2.5) -> ()  [unwired: 1 out]
  n66 = call <vilib>:"Square Waveform.vi"("offset"=0.0, "sampling info"=w73, "reset signal"=TRUE, "amplitude"=0.0, "frequency"=10.0) -> ("signal out"=w101:waveform(dbl))  [unwired: 5 in, 1 out]
  n67 = call <vilib>:"Square Waveform.vi"("offset"=0.0, "sampling info"=w40, "reset signal"=TRUE, "amplitude"=0.0, "frequency"=10.0) -> ("signal out"=w47:waveform(dbl))  [unwired: 5 in, 1 out]
  n68 = call-poly <vilib>:"Append Waveforms.vi"("waveform B"=w101, "waveform A"=w34) -> ("waveform out"=w46:waveform(dbl))  [unwired: 8 in, 1 out]
  n69 = for {
    N: w75 -> [_]
    tunnel: w46 -> [w163]
    shift-right: [w161] -> w38
    shift-left: w47 -> [w162]
    n70 = call-poly <vilib>:"Append Waveforms.vi"("waveform B"=w163, "waveform A"=w162) -> ("waveform out"=w161:waveform(dbl))  [unwired: 8 in, 1 out]
  }
  n71 = call <vilib>:"Square Waveform.vi"("offset"=0.0, "sampling info"=w72, "reset signal"=TRUE, "amplitude"=0.0, "frequency"=10.0) -> ("signal out"=w43:waveform(dbl))  [unwired: 5 in, 1 out]
  n72 = call-poly <vilib>:"Append Waveforms.vi"("waveform B"=w43, "waveform A"=w38) -> ("waveform out"=w36:waveform(dbl))  [unwired: 8 in, 1 out]
  n73 = call "XYWaveform.vi"("XYWaveformIN"=w13) -> ("XYWaveformOut"=w33:waveform(dbl))  [unwired: 10 in]
  n74 = call "XYWaveform.vi"("XYWaveformIN"=w12) -> ("XYWaveformOut"=w32:waveform(dbl))  [unwired: 10 in]
  n75 = call "XYWaveform.vi"("XYWaveformIN"=w24) -> ("XYWaveformOut"=w29:waveform(dbl))  [unwired: 10 in]
  n76 = Bundle By Name(cluster="SetupInfo_IN", "AnalogWaveform.Bi-lateral Galvo XY stand waveform"=w66, "AnalogWaveform.Bi-lateral Galvo XY OG waveform"=w127, "AnalogWaveform.Frontal Galvo XY OG waveform"=w123, "AnalogWaveform.Frontal Galvo XY stand waveform"=w120, "AnalogWaveform.Bi-lateral Galvo Z stand waveform"=w13, "AnalogWaveform.Frontal Galvo Z stand waveform"=w12, "AnalogWaveform.Detection objective stand waveform"=w24, "AnalogWaveform.sCMOS stand waveform"=w31, "AnalogWaveform.sCMOS blank waveform"=w114, "AnalogWaveform.PFI 0 clock stand waveform"=w113, "AnalogWaveform.AOM stand waveform"=w27, "DigitalWaveform.Plane Indexing"=w59, "AnalogWaveform.Bi-lateral Galvo Z OG waveform"=w61, "AnalogWaveform.Frontal Galvo Z OG waveform"=w60, "AnalogWaveform.Detection objective OG waveform"=w48, "AnalogWaveform.sCMOS OG waveform"=w36, "DigitalWaveform.Plane indexing P0.5 OG"=w70, "AnalogWaveform.PFI 0 clock OG wavee"=w69, "AnalogWaveform.AOM OG waveform"=w68, "AnalogWaveform.Bi-lateral Galvo Z XY"=w33, "AnalogWaveform.Frontal Galvo Z XY"=w32, "AnalogWaveform.sCMOS Trigger XY"=w30, "AnalogWaveform.Detection objective XY"=w29, "AnalogWaveform.AOM XY"=w28) -> (→"SetupInfo_OUT":T1)
  "error out" <- "error in (no error)"
